vi "Plot Label NumToString.vi"(0 "Digit Type":i32, 1 "Hide trailing zeros":bool, 5 "just/pad":i32(ring) items=["Pad with spaces on left", "Pad with spaces on right", "Pad with zeros on left"], 7 "Minimum Field Width":i32, 9 "Digits of Precision":i32, 11 "Numeric Format":i32, 12 "exponent":bool) -> (8 "Format String":string)   [LabVIEW 2020, in "3D Plot.lvclass"]
uses:
  3D Plot.lvclass
panel:
  # "0 = <no modifiers>\n1 = -\n2 = 0"
  # "0 = Left Justify\n1 = Right Justify"
  # "0 = Pad using zeros\n1 = Pad using spaces"
  # "Corresponds to the listbox on the property page \n0 = Floating Point   f\n1 = Scientific   e\n2 = Automatic   g\n3 = SI   p\n4 = unused\n5 = decimal\n6 = Hex     x\n7 = Oct      o\n8 = Bin    b"
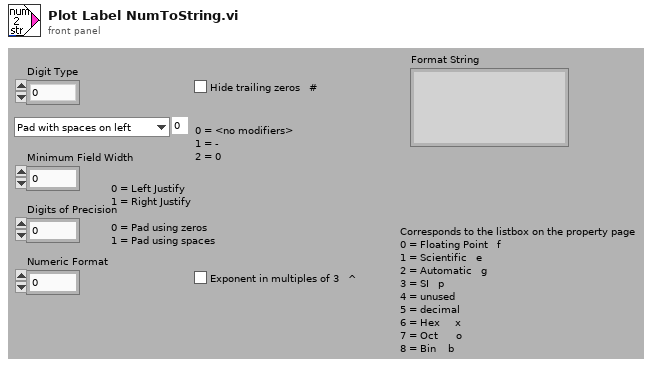
[diagram p1: front panel]
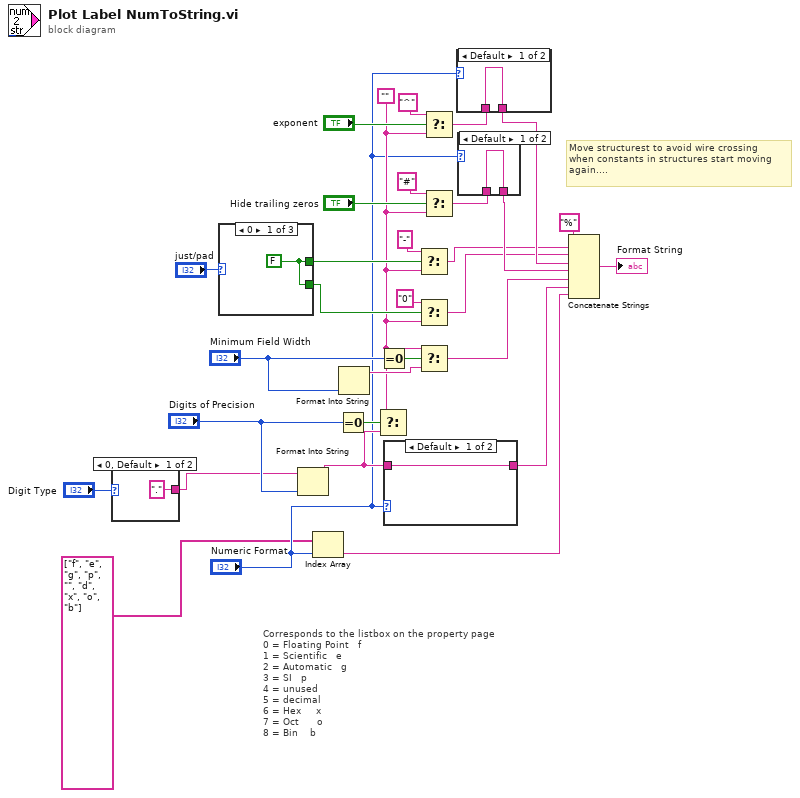
[diagram p0: block diagram]
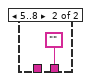
[diagram p2: hidden frame]
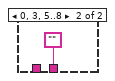
[diagram p3: hidden frame]
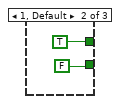
[diagram p4: hidden frame]
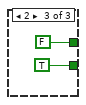
[diagram p5: hidden frame]
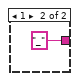
[diagram p6: hidden frame]
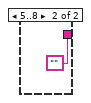
[diagram p7: hidden frame]
diagram:
  w10 = ""
  # "Move structurest to avoid wire crossing\nwhen constants in structures start moving\nagain...."
  # "Corresponds to the listbox on the property page \n0 = Floating Point   f\n1 = Scientific   e\n2 = Automatic   g\n3 = SI   p\n4 = unused\n5 = decimal\n6 = Hex     x\n7 = Oct      o\n8 = Bin    b"
  n1 = case shown="0, Default" "Digit Type" {
    tunnel: ["." ("Input String") "_" ("Input String")] -> w18
    frame 0, Default {
    }
    frame 1 {
    }
  }
  n2 = case shown="0" "just/pad" {
    tunnel: [w34 TRUE FALSE] -> w16
    tunnel: [w34 FALSE TRUE] -> w15
    frame 0 {
      w34 = FALSE
    }
    frame 1, Default {
    }
    frame 2 {
    }
  }
  n3 = Format Into String(initial string=w18, "Digits of Precision") -> (resulting string=w20:string)  [unwired: 2 in, 1 out]
  n4 = Index Array(array=string[] ["f", "e", "g", "p", "", "d", "x", "o", "b"] ("formats"), index="Numeric Format") -> (element=w28:string)
  n5 = Equal To 0?(x="Digits of Precision") -> (x = 0?=w27:bool)
  n6 = Format Into String("Minimum Field Width") -> (resulting string=w30:string)  [unwired: 3 in, 1 out]
  n7 = Select(t=w10, s=w27, f=w20) -> ()  [unwired: 1 out]
  n8 = Equal To 0?(x="Minimum Field Width") -> (x = 0?=w31:bool)
  n9 = case shown="Default" "Numeric Format" {
    tunnel: w20 -> [w39 _]
    tunnel: [w39 ""] -> w21
    frame Default {
    }
    frame 5..8 {
    }
  }
  n10 = Select(t="-" ("Input String"), s=w16, f=w10) -> (s? t:f=w3:string)
  n11 = Select(t="0" ("Input String"), s=w15, f=w10) -> (s? t:f=w2:string)
  n12 = Select(t=w10, s=w31, f=w30) -> (s? t:f=w29:string)
  n13 = Select(t="^" ("Input String"), s="exponent", f=w10) -> (s? t:f=w8:string)
  n14 = Select(t="#" ("Input String"), s="Hide trailing zeros", f=w10) -> (s? t:f=w6:string)
  n15 = case shown="Default" "Numeric Format" {
    tunnel: w8 -> [w41 _]
    tunnel: [w41 ""] -> w4
    frame Default {
    }
    frame 0, 3, 5..8 {
    }
  }
  n16 = case shown="Default" "Numeric Format" {
    tunnel: w6 -> [w43 _]
    tunnel: [w43 ""] -> w5
    frame Default {
    }
    frame 5..8 {
    }
  }
  n17 = Concatenate Strings("%" ("Substring"), w3, w2, w4, w5, w29, w21, w28) -> (→"Format String":string)
